vi "ImportStimuli.vi"(8 "error in (no error)":errorcluster, 9 "stimulus Description":string[](array[string]), 10 "stim_idx":dbl[](array[numeric]), 11 "Acquisition in":refnum<class "Acquisition.lvclass">) -> (0 "error out":errorcluster, 3 "Acquisition out":refnum<class "Acquisition.lvclass">)   [LabVIEW 2014, in "Acquisition.lvclass"]
uses:
  Acquisition.lvclass
  Acquisition.lvclass/Acquisition.ctl
  Database/Database.lvclass
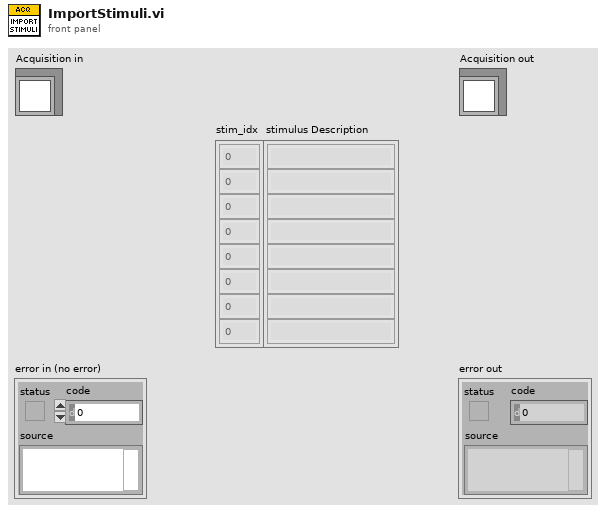
[diagram p1: front panel]
types:
  T1 = cluster{"mouse_id":dbl, "session_timestamp":string, "stimulus_index":dbl, "stimulus_description":string}
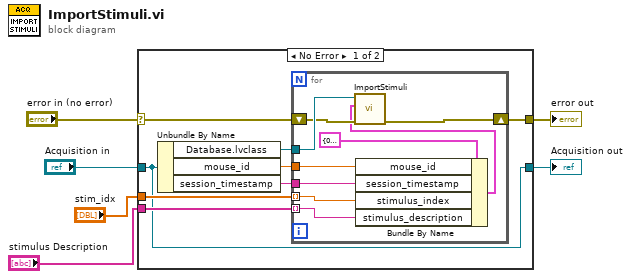
[diagram p0: block diagram]
diagram:
  n1 = case shown="No Error" "error in (no error)" {
    selector: "error in (no error)" -> [w8 w25]
    tunnel: [w7 w25] -> w5
    tunnel: [w12 w24] -> w3
    tunnel: "Acquisition in" -> [w12 w24]
    tunnel: "stimulus Description" -> [w14 _]
    tunnel: "stim_idx" -> [w13 _]
    frame No Error {
      n2 = Unbundle By Name(w12) -> ("Database.lvclass"=w11:refnum<class "Database.lvclass">, "mouse_id"=w9:dbl, "session_timestamp"=w10:string)
      n3 = for {
        tunnel: w14 -> [w21] mode=indexing
        tunnel: w13 -> [w20] mode=indexing
        tunnel: w11 -> [w23]
        tunnel: w10 -> [w19]
        tunnel: w9 -> [w18]
        shift-right: [w16] -> w7
        shift-left: w8 -> [w17]
        n4 = Bundle By Name(cluster=T1 {"mouse_id"=0.0, "session_timestamp"="2016-04-18 10:52:44", "stimulus_index"=0.0, "stimulus_description"=""} ("Tuple"), "mouse_id"=w18, "session_timestamp"=w19, "stimulus_index"=w20, "stimulus_description"=w21) -> (w15:T1)
        n5 = call-dynamic "ImportStimuli.vi"("error in (no error)"=w17, "Tuple"=w15, "Database in"=w23) -> ("error out"=w16:errorcluster)  [unwired: 7 in, 1 out]
      }
    }
    frame Error {
    }
  }
  "error out" <- w5
  "Acquisition out" <- w3
